vi "PAN_StartStartCommMod.vi"(4 "start":bool=TRUE, 6 "running":bool, 7 "ModPath":path, 8 "error in (no error)":errorcluster, 9 "openpanel":bool, 10 "commod":string) -> (0 "error out":errorcluster, 2 "response":string)   [LabVIEW 2016]
uses:
  <vilib>/Utility/error.llb/DialogType.ctl
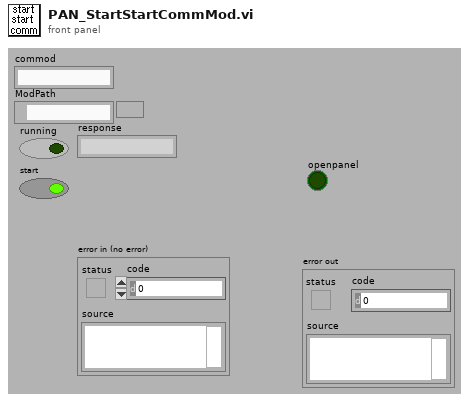
[diagram p1: front panel]
types:
  T1 = typedef "DialogType.ctl" = u16
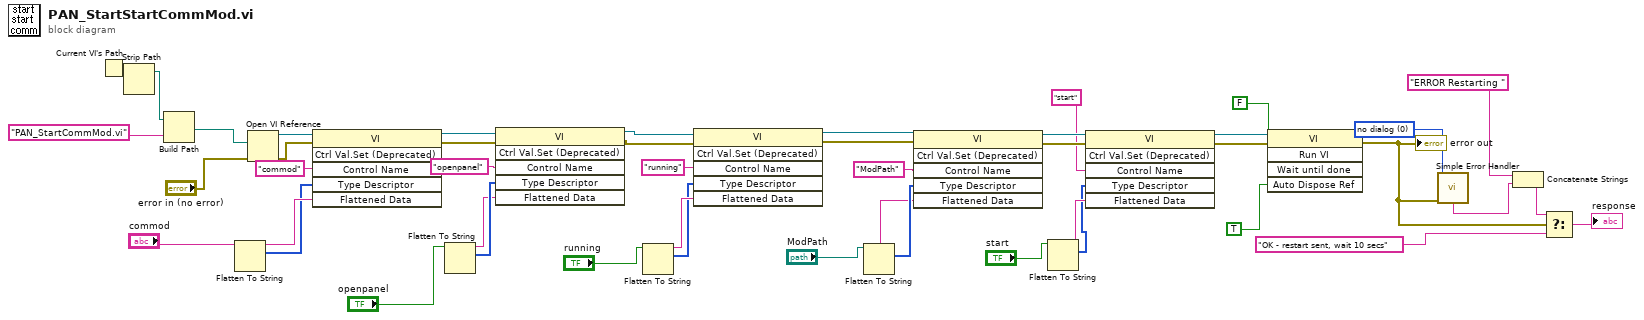
[diagram p0: block diagram]
diagram:
  w13 = T1 0 items=["no dialog", "OK message", "continue or stop message", "OK message + warnings", "continue/stop + warnings"] ("type of dialog (OK msg:1)")
  n1 = Current VI's Path() -> (path=w11:path)
  n2 = Strip Path(path=w11) -> (stripped path=w10:path)  [unwired: 1 out]
  n3 = Build Path(base path=w10, name or relative path="PAN_StartCommMod.vi" ("string")) -> (appended path=w46:path)
  n4 = Flatten To String(anything="commod") -> (data string=w36:string, type string=w35:i16[])  [unwired: 1 in, 3 out]
  n5 = Open VI Reference(vi path=w46, error in (no error)="error in (no error)") -> (vi reference=w40:refnum<vi>, error out=w39:errorcluster)  [unwired: 4 out]
  n6 = invoke class="VI" method="Ctrl Val.Set (Deprecated)"(reference=w40, error in=w39, "Control Name"="commod", "Type Descriptor"=w35, "Flattened Data"=w36) -> (reference out=w34:refnum<vi>, error out=w33:errorcluster)  [unwired: 1 in, 4 out]
  n7 = Flatten To String(anything="openpanel") -> (data string=w30:string, type string=w31:i16[])  [unwired: 1 in, 3 out]
  n8 = invoke class="VI" method="Ctrl Val.Set (Deprecated)"(reference=w34, error in=w33, "Control Name"="openpanel", "Type Descriptor"=w31, "Flattened Data"=w30) -> (reference out=w25:refnum<vi>, error out=w24:errorcluster)  [unwired: 1 in, 4 out]
  n9 = Flatten To String(anything="running") -> (data string=w27:string, type string=w26:i16[])  [unwired: 1 in, 3 out]
  n10 = invoke class="VI" method="Ctrl Val.Set (Deprecated)"(reference=w25, error in=w24, "Control Name"="running", "Type Descriptor"=w26, "Flattened Data"=w27) -> (reference out=w22:refnum<vi>, error out=w21:errorcluster)  [unwired: 1 in, 4 out]
  n11 = Flatten To String(anything="ModPath") -> (data string=w43:string, type string=w44:i16[])  [unwired: 1 in, 3 out]
  n12 = invoke class="VI" method="Ctrl Val.Set (Deprecated)"(reference=w22, error in=w21, "Control Name"="ModPath", "Type Descriptor"=w44, "Flattened Data"=w43) -> (reference out=w8:refnum<vi>, error out=w6:errorcluster)  [unwired: 1 in, 4 out]
  n13 = Flatten To String(anything="start") -> (data string=w2:string, type string=w1:i16[])  [unwired: 1 in, 3 out]
  n14 = invoke class="VI" method="Ctrl Val.Set (Deprecated)"(reference=w8, error in=w6, "Control Name"="start", "Type Descriptor"=w1, "Flattened Data"=w2) -> (reference out=w7:refnum<vi>, error out=w5:errorcluster)  [unwired: 1 in, 4 out]
  n15 = invoke class="VI" method="Run VI"(reference=w7, error in=w5, "Wait until done"=FALSE ("Wait Until Done"), "Auto Dispose Ref"=TRUE ("Auto Dispose Reference")) -> (error out=w17:errorcluster)  [unwired: 1 in, 4 out]
  "error out" <- w17
  n16 = call <vilib>:"Simple Error Handler.vi"("type of dialog (OK msg:1)"=w13, "error in (no error)"=w17) -> ("message"=w14:string)  [unwired: 7 out]
  n17 = Concatenate Strings("ERROR Restarting " ("string"), w14) -> (w15:string)
  n18 = Select(t=w15, s=w17, f="OK - restart sent, wait 10 secs" ("response")) -> (s? t:f=→"response":string)
